vi "S2DS_Writing buffer to file.vi"(0 "Data save info (in)":T1={"File path"=path "", "Header"="", "File name"="", "False channel"=[], "Channel names"=[], "Buffer size"=0, "Format"="%.6f"}, 2 "Data array in":dbl[][](array[numeric]), 3 "Buffer length":i32) -> (6 "Data save info (out)":T1={"File path"=path "", "Header"="", "File name"="", "False channel"=[], "Channel names"=[], "Buffer size"=0, "Format"="%.6f"}, 8 "Data array out":dbl[][](array[numeric]), 9 "Buffer length out":i32)   [LabVIEW 2025]
uses:
  TYPE DEFS/S2DS_Data saving info.ctl
  <vilib>/Utility/file.llb/Write To Spreadsheet File (DBL).vi
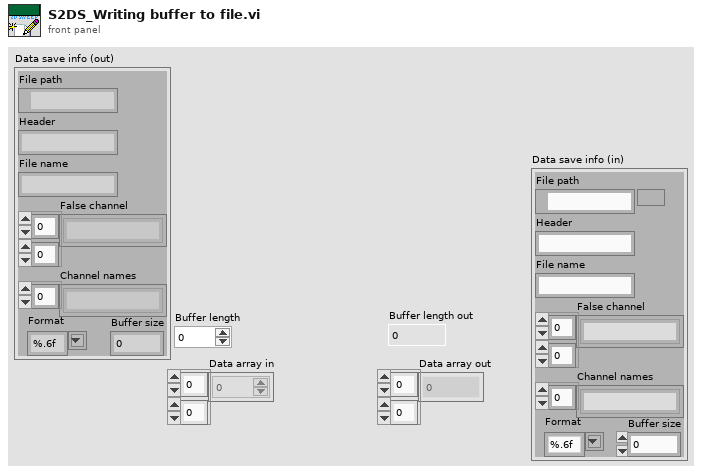
[diagram p1: front panel]
types:
  T1 = typedef "S2DS_Data saving info.ctl" = cluster{"File path":path, "Header":string, "File name":string, "False channel":string[][], "Channel names":string[], "Buffer size":i32, "Format":string}
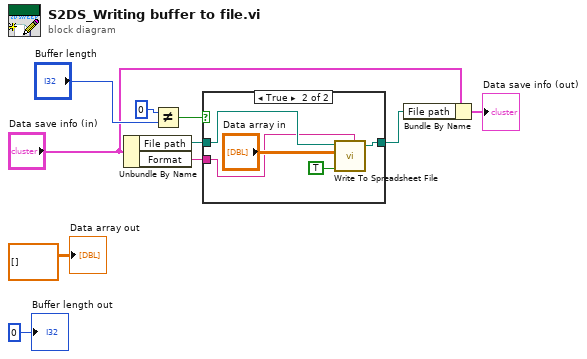
[diagram p0: block diagram]
diagram:
  n1 = Unbundle By Name("Data save info (in)") -> ("File path"=w5:path, "Format"=w1:string)
  n2 = Not Equal?(x=0, y="Buffer length") -> (x != y?=w7:bool)
  n3 = case shown="True" w7 {
    tunnel: [w11 w14] -> w3
    tunnel: w5 -> [w11 w13]
    tunnel: w1 -> [_ w12]
    frame False {
    }
    frame True {
      n4 = call-poly <vilib>:"Write To Spreadsheet File.vi"("format (%.3f)"=w12, "append to file? (new file:F)"=TRUE, "2D data"="Data array in", "file path (dialog if empty)"=w13) -> ("new file path (Not A Path if cancelled)"=w14:path)  [unwired: 4 in]
    }
  }
  n5 = Bundle By Name(cluster="Data save info (in)", "File path"=w3) -> (→"Data save info (out)":T1)
  "Data array out" <- dbl[][] [] ("Data array out")
  "Buffer length out" <- 0 ("Buffer length out")
